vi "J1939 Message TP.CM CTS.vi"(0 "PGN":u32 format="%.0x", 1 "Source Address":u8=27, 2 "Destination Address":u8, 5 "Number of Packets to Send":u8, 7 "Next Packet to Send":u8, 11 "error in (no error)":errorcluster) -> (4 "Arb ID":u32 format="%.0x", 8 "Data":u8[](array[numeric]), 15 "error out":errorcluster)   [LabVIEW 2013, in "J1939.lvlib"]
uses:
  J1939.lvlib
  API Types/PGN Fields Cluster.ctl
  Frame Conversion/Convert J1939 ID to CAN Arb ID.vi
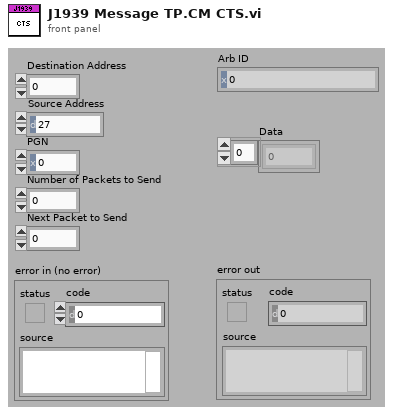
[diagram p1: front panel]
types:
  T1 = typedef "J1939.lvlib/PGN Fields Cluster.ctl" = cluster{"Reserved Bit":u8, "Data page":u8, "PDU Format":u8, "PDU Specific":u8}
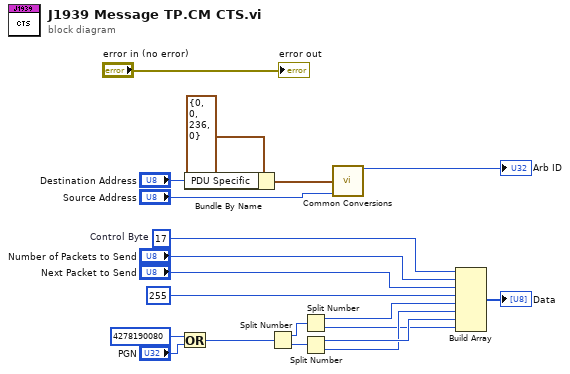
[diagram p0: block diagram]
diagram:
  w8 = u8 17  # Control Byte
  n1 = Or(x=u32 4278190080, y="PGN") -> (x .or. y?=w7:u32)
  n2 = Bundle By Name(cluster=T1 {"Reserved Bit"=0, "Data page"=0, "PDU Format"=236, "PDU Specific"=0} ("PGN Fields"), "PDU Specific"="Destination Address") -> (w15:T1)
  n3 = Split Number(x=w7) -> (hi(x)=w5:u16, lo(x)=w6:u16)
  n4 = Split Number(x=w5) -> (hi(x)=w4:u8, lo(x)=w1:u8)
  n5 = Split Number(x=w6) -> (hi(x)=w3:u8, lo(x)=w2:u8)
  n6 = call-poly "Common Conversions.vi"("PGN Fields"=w15, "Source Address"="Source Address") -> ("ID"=→"Arb ID":u32)  [unwired: 3 in, 10 out]
  n7 = Build Array(w8, "Number of Packets to Send", "Next Packet to Send", u8 255, w4, w2, w3, w1) -> (→"Data":u8[])
  "error out" <- "error in (no error)"
